vi "CMN_FileTPL2Array.vi"(7 "mext":bool, 8 "error in (no error)":errorcluster, 9 "number of Extensions":u16, 10 "filename":path) -> (0 "error out":errorcluster, 1 "number of keys":i32[](array[numeric]), 2 "flat keys":string[][](array[string]), 3 "Keys":string[][][](array[string]), 4 "Extensions":i32[][](array[numeric]))   [LabVIEW 2016]
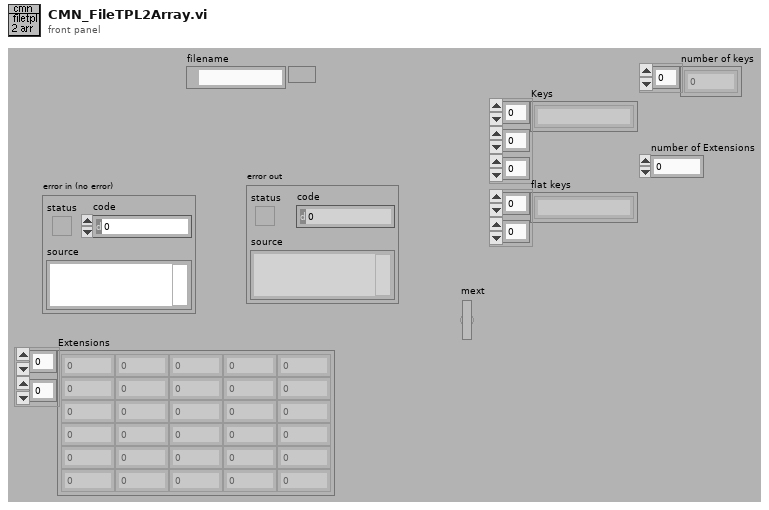
[diagram p1: front panel]
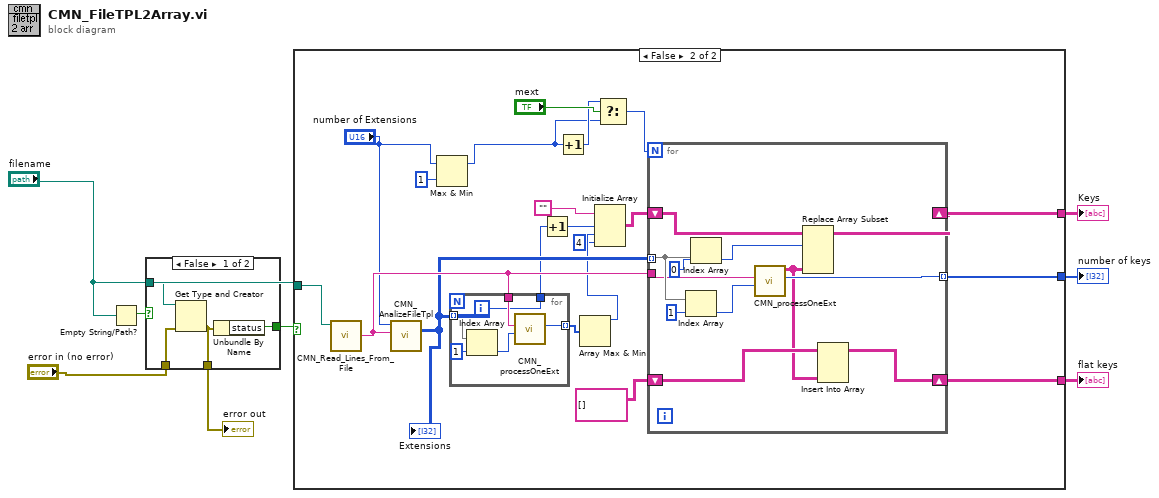
[diagram p0: block diagram]
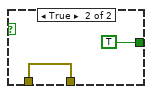
[diagram p2: hidden frame]
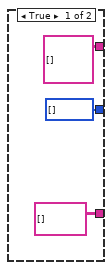
[diagram p3: hidden frame]
diagram:
  n1 = Empty String/Path?(string/path="filename") -> (empty?=w7:bool)
  n2 = case shown="False" w7 {
    tunnel: [w12 TRUE ("status")] -> w8
    tunnel: "filename" -> [w11 _]
    tunnel: "error in (no error)" -> [w10 w13]
    tunnel: [w9 w13] -> w1
    frame False {
      n3 = Get Type and Creator(4:w10, 7:w11) -> (0:w9:errorcluster)  [unwired: 3 out]
      n4 = Unbundle By Name(w9) -> ("status"=w12:bool)
    }
    frame True {
    }
  }
  "error out" <- w1
  n5 = case shown="False" w8 {
    tunnel: "filename" -> [_ w35]
    tunnel: [string[][][] [] w37] -> w5
    tunnel: [i32[] [] w36] -> w3
    tunnel: [string[][] [] w33] -> w4
    frame True {
      (unwired) string[][] []
      (unwired) 0
    }
    frame False {
      n6 = call "CMN_Read_Lines_From_File.vi"("file path"=w35) -> ("line string"=w32:string)  [unwired: 1 in, 7 out]
      n7 = call "CMN_AnalizeFileTpl.vi"("line string"=w32, "number of Extensions"="number of Extensions") -> ("Extensions"=w30:i32[][])  [unwired: 9 out]
      "Extensions" <- w30
      n8 = Max & Min(x="number of Extensions", y=u16 1) -> (max(x,y)=w19:u16)  [unwired: 1 out]
      n9 = for {
        tunnel: w30 -> [w43] mode=indexing
        tunnel: w32 -> [w41]
        tunnel: [w40] -> w31 mode=indexing
        tunnel: [w38] -> w28
        i -> [w38]
        n10 = Index Array(array=w43, index=1) -> (element=w42:i32)
        n11 = call "CMN_processOneExt.vi"("starting line"=w42, "str in"=w41) -> ("number of keywords found"=w40:i32)  [unwired: 3 in, 6 out]
      }
      n12 = Increment(x=w28) -> (x+1=w24:i32)
      n13 = Increment(x=w19) -> (x+1=w20:u16)
      n14 = Array Max & Min(array=w31) -> (max value=w27:i32)  [unwired: 3 out]
      n15 = Initialize Array("", w24, w27, 4 ("dimension size")) -> (w25:string[][][])
      n16 = Select(t=w20, s="mext", f=w19) -> (s? t:f=w18:u16)
      n17 = for {
        N: w18 -> [_]
        shift-right: [w48] -> w37
        shift-left: w25 -> [w50]
        tunnel: w30 -> [w55] mode=indexing
        tunnel: w32 -> [w52]
        tunnel: [w49] -> w36 mode=indexing
        shift-right: [w45] -> w33
        shift-left: string[][] [] -> [w46]
        n18 = Index Array(array=w55, index=1 ("Index")) -> (element=w51:i32)
        n19 = Index Array(array=w55, index=0 ("Index")) -> (element=w47:i32)
        n20 = call "CMN_processOneExt.vi"("starting line"=w51, "str in"=w52) -> ("number of keywords found"=w49:i32, "HdrInfo"=w44:string[][])  [unwired: 3 in, 5 out]
        n21 = Replace Array Subset(array=w50, new element=w44, index (dim 0)=w47) -> (w48:string[][][])  [unwired: 2 in]
        n22 = Insert Into Array(array=w46, new element=w44) -> (w45:string[][])  [unwired: 2 in]
      }
    }
  }
  "Keys" <- w5
  "flat keys" <- w4
  "number of keys" <- w3
